vi "ProdaNG.CreateProduct.vi"(8 "error in (no error)":errorcluster, 9 "serialNumber":string, 10 "ID":T3, 11 "dbHandle":i32) -> (0 "error out":errorcluster, 1 "Product out":T2, 2 "Status":T1, 3 "dbHandle out":i32)   [LabVIEW 2016]
doc: "This function returns a product structure for a product, which is identified by a part and a serial number.\nImportant information: The field 'individual' was taken over from the field 'allgemein' of the legacy data directly. Because of this most products have the value 0 further on and only a few the value 1. \nParameter:\nhandle is an Integer, which is returned by the function Login() at the creation of a new connection.\nwabcoPartId is the Id of the part.\nserialNumber is the serial number of the product for the part above.\nproduct is a pointer on a product structure, which is filled if the returncode is 0. The structure must be defined in the calling program.\n\nReturncodes:\n0 No error\n< 0 ORACLE Error code\n6 (ERROR_INVALID_HANDLE) in case of an invalid handle\n1403 Record does not exist"
uses:
  Controls/ProdaNG.Identification.ctl
  Controls/ProdaNG.Product.ctl
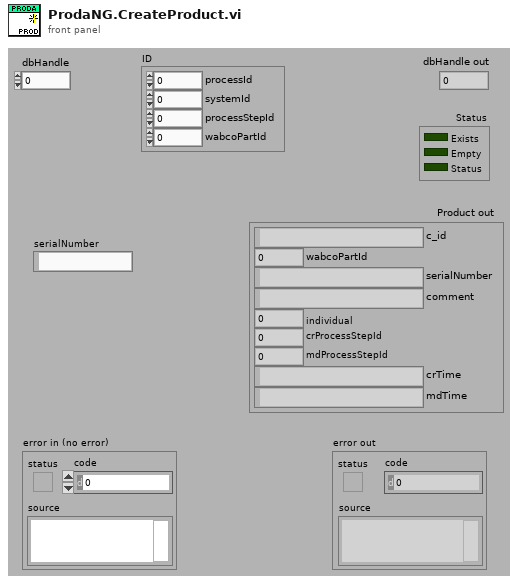
[diagram p1: front panel]
types:
  T1 = cluster{"Exists":bool, "Empty":bool, "Status":bool}
  T2 = typedef "ProdaNG.Product.ctl" = cluster{"c_id":string, "wabcoPartId":i32, "serialNumber":string, "comment":string, "individual":i32, "crProcessStepId":i32, "mdProcessStepId":i32, "crTime":string, "mdTime":string}
  T3 = typedef "ProdaNG.Identification.ctl" = cluster{"processId":i32, "systemId":i32, "processStepId":i32, "wabcoPartId":i32}
  T4 = typedef "ProdaNG.ProcessResult.ctl" = cluster{"c_id":string, "productId":string, "processId":i32, "statusId":i32, "startTime":string, "endTime":string}
  T5 = typedef "ProdaNG.ProcessStepResult.ctl" = cluster{"c_id":string, "processResultId":string, "processStepId":i32, "statusId":i32, "operatorId":i32, "startTime":string, "endTime":string}
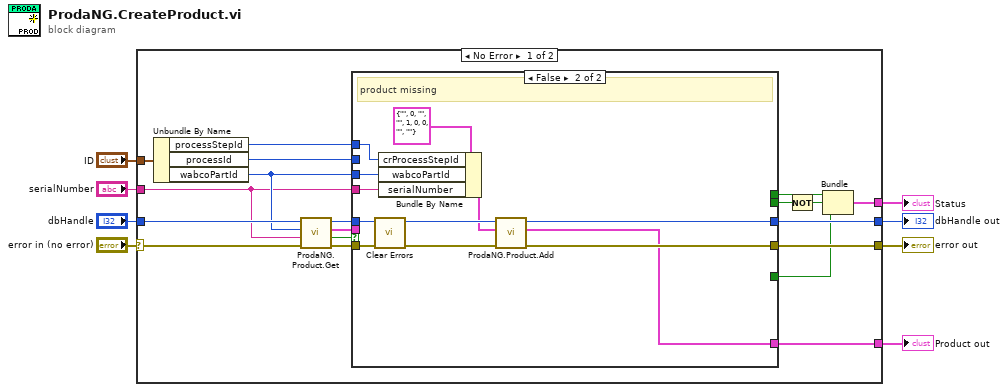
[diagram p0: block diagram]
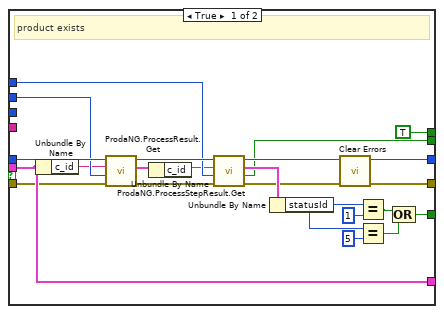
[diagram p2: hidden frame]
diagram:
  n1 = case shown="No Error" "error in (no error)" {
    selector: "error in (no error)" -> [w27 w62]
    tunnel: [w24 w62] -> w7
    tunnel: "dbHandle" -> [w20 w61]
    tunnel: [w21 w61] -> w5
    tunnel: "serialNumber" -> [w11 _]
    tunnel: "ID" -> [w19 _]
    tunnel: [w15 _] -> w2
    tunnel: [w12 _] -> w1
    frame No Error {
      n2 = Unbundle By Name(w19) -> ("processStepId"=w17:i32, "processId"=w16:i32, "wabcoPartId"=w18:i32)
      n3 = call "ProdaNG.Product.Get.vi"("error in (no error)"=w27, "serialNumber"=w11, "wabcoPartId"=w18, "dbHandle"=w20) -> ("error out"=w26:errorcluster, "found"=w25:bool, "Product"=w23:T2, "dbHandle out"=w22:i32)  [unwired: 4 in]
      n4 = case shown="False" w25 {
        tunnel: w26 -> [w45 w60]
        tunnel: [w41 w57] -> w24
        tunnel: [w28 _] -> w14
        tunnel: w23 -> [w46 _]
        tunnel: w22 -> [w44 w58]
        tunnel: [w49 w54] -> w21
        tunnel: [w39 _] -> w9
        tunnel: w18 -> [_ w56]
        tunnel: w11 -> [_ w55]
        tunnel: w17 -> [w31 w50]
        tunnel: w16 -> [w32 _]
        tunnel: [w46 w53] -> w15
        tunnel: [TRUE _] -> w13
        frame True {
          # "product exists"
          n5 = Unbundle By Name(w46) -> ("c_id"=w29:string)
          n6 = call "ProdaNG.ProcessResult.Get.vi"("error in (no error)"=w45, "processId"=w32, "productId"=w29, "dbHandle"=w44) -> ("error out"=w34:errorcluster, "ProcessResult"=w43:T4, "dbHandle out"=w42:i32)  [unwired: 4 in, 1 out]
          n7 = Unbundle By Name(w43) -> ("c_id"=w30:string)
          n8 = call "ProdaNG.ProcessStepResult.Get.vi"("error in (no error)"=w34, "processStepId"=w31, "processResultId"=w30, "dbHandle"=w42) -> ("error out"=w35:errorcluster, "Found"=w28:bool, "ProcessStepResult"=w36:T5, "dbHandle out"=w49:i32)  [unwired: 4 in]
          n9 = Unbundle By Name(w36) -> ("statusId"=w37:i32)
          n10 = call <vilib>:"Clear Errors.vi"("error in (no error)"=w35) -> ("error out"=w41:errorcluster)  [unwired: 5 in, 1 out]
          n11 = Equal?(x=w37, y=1) -> (x = y?=w48:bool)
          n12 = Equal?(x=w37, y=5) -> (x = y?=w38:bool)
          n13 = Compound Arithmetic op=OR(w48, w38) -> (w39:bool)
        }
        frame False {
          # "product missing"
          n14 = call <vilib>:"Clear Errors.vi"("error in (no error)"=w60) -> ("error out"=w59:errorcluster)  [unwired: 5 in, 1 out]
          n15 = Bundle By Name(cluster=T2 {"c_id"="", "wabcoPartId"=0, "serialNumber"="", "comment"="", "individual"=1, "crProcessStepId"=0, "mdProcessStepId"=0, "crTime"="", "mdTime"=""} ("Product"), "crProcessStepId"=w50, "wabcoPartId"=w56, "serialNumber"=w55) -> (w51:T2)
          n16 = call "ProdaNG.Product.Add.vi"("error in (no error)"=w59, "Product"=w51, "dbHandle"=w58) -> ("error out"=w57:errorcluster, "Product out"=w53:T2, "dbHandle"=w54:i32)  [unwired: 6 in]
        }
      }
      n17 = Not(x=w14) -> (.not. x?=w10:bool)
      n18 = Bundle(w13, w10, w9) -> (w12:cluster{bool, bool, bool})  [unwired: 1 in]
    }
    frame Error {
    }
  }
  "error out" <- w7
  "dbHandle out" <- w5
  "Product out" <- w2
  "Status" <- w1
